vi "Initialize.vi"(8 "error in":errorcluster, 11 "TCP master in":refnum<class "TCP Master.lvclass">) -> (0 "error out":errorcluster, 3 "TCP master out":refnum<class "TCP Master.lvclass">)   [LabVIEW 2021, in "TCP Master.lvclass"]
doc: "Opens a TCP connection to the address and port stored in the class."
uses:
  TCP Master.lvclass
  D:/my_projects/projects/Algorithms/Labview/21/Modbus_v121c/Network Protocol/Network Master/Network Master.lvclass
  Network Master.lvclass/Network Master.ctl
  Transmission Data Unit/Transmission Data Unit.lvclass
  Network Master.lvclass
  TCP Master.lvclass/TCP Master.ctl
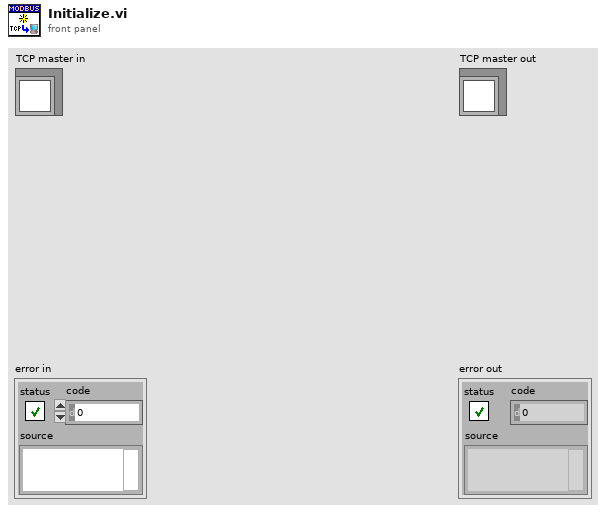
[diagram p1: front panel]
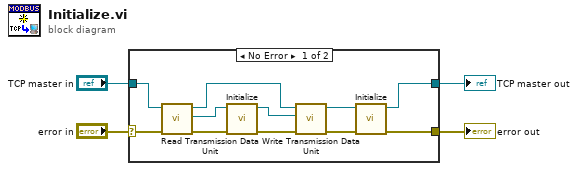
[diagram p0: block diagram]
diagram:
  n1 = case shown="No Error" "error in" {
    selector: "error in" -> [w13 w17]
    tunnel: "TCP master in" -> [w15 w16]
    tunnel: [w9 w16] -> w3
    tunnel: [w10 w17] -> w2
    frame No Error {
      n2 = call "Read Transmission Data Unit.vi"("error in (no error)"=w13, "Network Master in"=w15) -> ("error out"=w8:errorcluster, "Transmission Data Unit"=w7:refnum<class "Transmission Data Unit.lvclass">, "Network Master out"=w14:refnum<class "TCP Master.lvclass">)  [unwired: 7 in]
      n3 = call-dynamic "Initialize.vi"("error in"=w8, "transmission data unit in"=w7) -> ("error out"=w6:errorcluster, "transmission data unit out"=w5:refnum<class "Transmission Data Unit.lvclass">)  [unwired: 8 in]
      n4 = call "Write Transmission Data Unit.vi"("error in (no error)"=w6, "Transmission Data Unit"=w5, "Network Master in"=w14) -> ("error out"=w12:errorcluster, "Network Master out"=w11:refnum<class "TCP Master.lvclass">)  [unwired: 7 in]
      n5 = call-parent "Initialize.vi"("error in"=w12, "Network Master in"=w11) -> ("error out"=w10:errorcluster, "Network Master out"=w9:refnum<class "TCP Master.lvclass">)  [unwired: 8 in]
    }
    frame Error {
    }
  }
  "error out" <- w2
  "TCP master out" <- w3
